vi "Error Handler.vi"(8 "error in":errorcluster, 11 "queue in":refnum<queue>) -> (0 "error out":errorcluster, 3 "queue out":refnum<queue>)   [LabVIEW 2024]
doc: "This subVI monitors the Error Cluster wire running through both the Producer and Consumer Loops. The moment an Error is detected in either loop this subVI sends a message to the Consumer Loop to shut down."
uses:
  Consumer Message.ctl
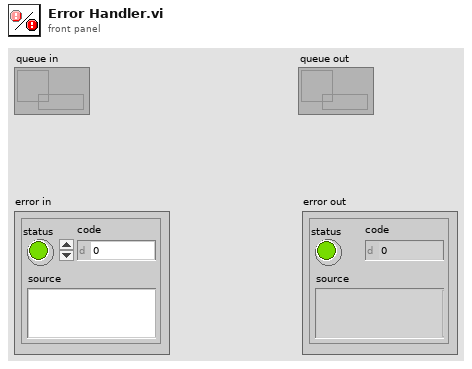
[diagram p1: front panel]
types:
  T1 = typedef "Consumer Message.ctl" = cluster{"Consumer State":string, "Boolean Data":bool, "Numeric Data":i32, "Error":errorcluster}
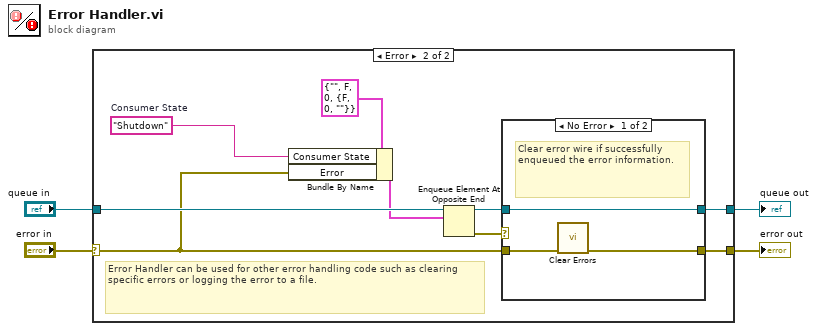
[diagram p0: block diagram]
diagram:
  n1 = case shown="Error" "error in" {
    selector: "error in" -> [w6 w10]
    tunnel: [w6 w13] -> w3
    tunnel: "queue in" -> [w5 w15]
    tunnel: [w5 w7] -> w1
    frame No Error {
    }
    frame Error {
      w11 = "Shutdown"  # Consumer State
      # "Error Handler can be used for other error handling code such as clearing specific errors or logging the error to a file."
      n2 = Bundle By Name(cluster=T1 {"Consumer State"="", "Boolean Data"=FALSE, "Numeric Data"=0, "Error"={"status"=FALSE, "code"=0, "source"=""}}, "Consumer State"=w11, "Error"=w10) -> (w14:T1)
      n3 = Enqueue Element At Opposite End(queue=w15, element=w14) -> (queue out=w8:refnum<queue>, error out=w9:errorcluster)  [unwired: 2 in, 1 out]
      n4 = case shown="No Error" w9 {
        selector: w9 -> [_ w20]
        tunnel: [w18 w20] -> w13
        tunnel: w10 -> [w17 _]
        tunnel: w8 -> [w16 w19]
        tunnel: [w16 w19] -> w7
        frame No Error {
          # "Clear error wire if successfully enqueued the error information."
          n5 = call <vilib>:"Clear Errors.vi"("error in (no error)"=w17) -> ("error out"=w18:errorcluster)  [unwired: 5 in, 1 out]
        }
        frame Error {
          # "If Queue function fails then pass the error out."
        }
      }
    }
  }
  "error out" <- w3
  "queue out" <- w1
